vi "Perform Action on Target.vi"(8 "error in":errorcluster, 9 "Input":variant, 10 "Task-Point Ident":string, 11 "Study Actor in":refnum<class "Study Actor.lvclass">) -> (0 "error out":errorcluster, 1 "Output":variant, 3 "Study Actor out":refnum<class "Study Actor.lvclass">)   [LabVIEW 2023, in "Study Actor.lvlib" / "Study Actor.lvclass"]
uses:
  Study Actor.lvclass
  Study Actor.lvclass/Study Actor.ctl
  <vilib>/ni/Actors/Network Endpoint Actors/Protocols/Network Stream Strategy/Network Stream Initiator/Network Stream Initiator.lvclass
  C:/Program Files/National Instruments/LabVIEW 2023/vi.lib/ni/Actors/Network Endpoint Actors/Protocols/Network Stream Strategy/Network Stream/Network Stream.lvclass
  Reply Protocol/Reply Protocol DataSocket/Reply Protocol DataSocket.lvclass
  <vilib>/ni/Actors/Network Endpoint Actors/Protocols/Network Stream Strategy/Network Stream/Network Stream.lvclass/Network Stream.ctl
  Reply Protocol/Reply Protocol DataSocket/Reply Protocol DataSocket.lvclass/Reply Protocol DataSocket.ctl
  MSS Target/IMSS Target Actor Messages/Perform Action Msg/Perform Action Msg.lvclass/Perform Action Msg.ctl
  MSS Target/IMSS Target Actor Messages/Perform Action Msg/Perform Action Msg.lvclass
  D:/git/DS-Reply-Msg/DS Reply Msg/DS Reply Msg.lvclass
  <vilib>/Utility/error.llb/Error Cluster From Error Code.vi
  DS-Reply-Msg/DS Reply Msg/Send Message and Wait for Response.vi
  <vilib>/ErrorRing/Error Ring.xnode
  <vilib>/ni/Actors/Network Endpoint Actors/Protocols/Network Stream Strategy/Network Stream/Network Stream.lvclass
  Reply Protocol Manager/Reply Protocol Manager.lvclass
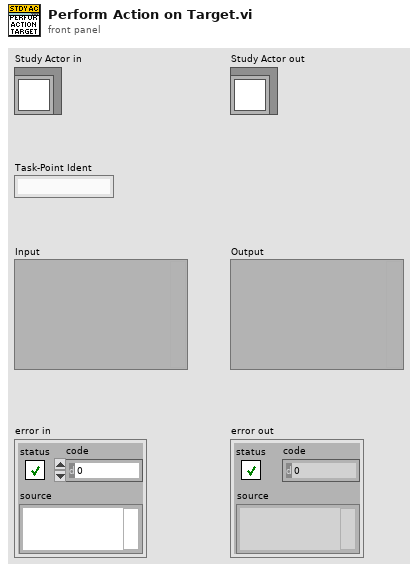
[diagram p1: front panel]
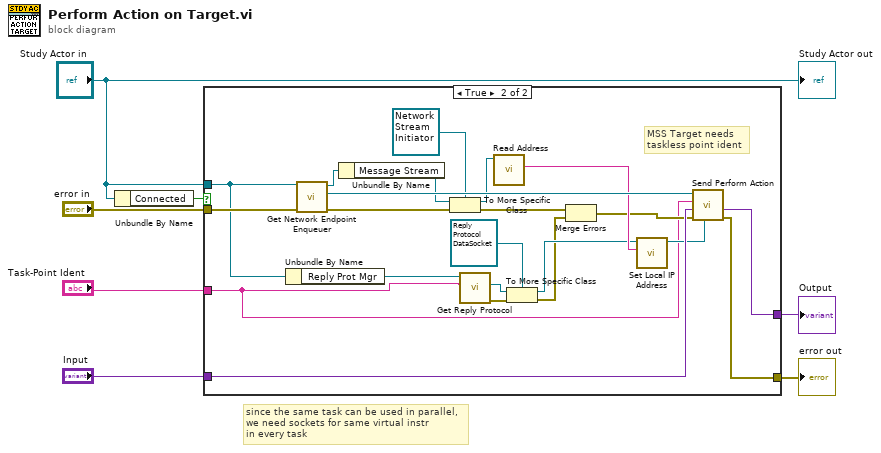
[diagram p0: block diagram]
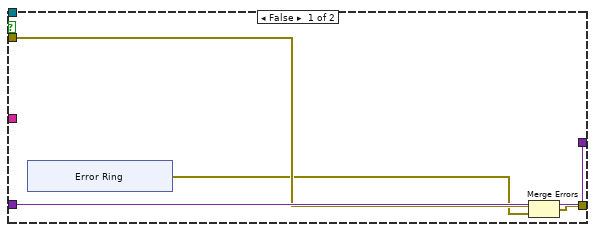
[diagram p2: hidden frame]
diagram:
  # "since the same task can be used in parallel,\nwe need sockets for same virtual instr\nin every task"
  n1 = Unbundle By Name("Study Actor in") -> ("Connected"=w7:bool)
  n2 = case shown="True" w7 {
    tunnel: "Study Actor in" -> [_ w26]
    tunnel: "error in" -> [w10 w38]
    tunnel: [w9 w35] -> w4
    tunnel: "Input" -> [w11 w36]
    tunnel: [w11 w34] -> w2
    tunnel: "Task-Point Ident" -> [_ w17]
    frame False {
      n3 = xnode "Error Ring"() -> ("error out"=w8:errorcluster)
      n4 = Merge Errors(w10, w8) -> (w9:errorcluster)
    }
    frame True {
      # "MSS Target needs\ntaskless point ident"
      n5 = Unbundle By Name(w26) -> ("Reply Prot Mgr"=w25:refnum<class "Reply Protocol Manager.lvclass">)
      n6 = call "Get Network Endpoint Enqueuer.vi"("error in"=w38, "Study Actor in"=w26) -> ("error out"=w18:errorcluster, "Network Endpoint Enqueuer"=w37:refnum<class "Message Enqueuer.lvclass">, "Study Actor out"=w33:refnum<class "Study Actor.lvclass">)  [unwired: 6 in, 1 out]
      n7 = Unbundle By Name(w33) -> ("Message Stream"=w32:refnum<class "Message Stream.lvclass">)
      n8 = To More Specific Class(target class=refnum<class "Network Stream Initiator.lvclass"> refnum ("Network Stream Initiator out"), reference=w32, error in=w18) -> (specific class reference=w30:refnum<class "Network Stream Initiator.lvclass">, error out=w29:errorcluster)
      n9 = call "Get Reply Protocol.vi"("Identifier"=w17, "reference in"=w25) -> ("Error Out"=w24:errorcluster, "Reply Protocol Base"=w23:refnum<class "Reply Protocol Base.lvclass">)  [unwired: 7 in, 1 out]
      n10 = call <vilib>:"Read Address.vi"("Network Stream in"=w30) -> ("Address"=w27:string)  [unwired: 10 in]
      n11 = To More Specific Class(target class=refnum<class "Reply Protocol DataSocket.lvclass"> refnum ("Reply Protocol DataSocket in"), reference=w23, error in=w24) -> (specific class reference=w21:refnum<class "Reply Protocol DataSocket.lvclass">, error out=w19:errorcluster)
      n12 = Merge Errors(w29, w19) -> (w20:errorcluster)
      n13 = call "Set Local IP Address.vi"("Local IP Address"=w27, "Reply Protocol DataSocket in"=w21) -> ("Reply Protocol DataSocket out"=w28:refnum<class "Reply Protocol DataSocket.lvclass">)  [unwired: 9 in]
      n14 = call "Send Perform Action.vi"("Reply Protocol DataSocket in"=w28, "error in"=w20, "Input"=w36, "Task-Point Ident"=w17, "Message Enqueuer"=w37) -> ("error out"=w35:errorcluster, "Output"=w34:variant)  [unwired: 3 in, 2 out]
    }
  }
  "error out" <- w4
  "Output" <- w2
  "Study Actor out" <- "Study Actor in"
